vi "Reset.vi"(10 "Index":i32, 11 "Variables in":refnum<class "Variables.lvclass">) -> (3 "Variables out":refnum<class "Variables.lvclass">)   [LabVIEW 2020, in "VolatusSeq.lvlib" / "Variables.lvclass"]
uses:
  Variables.lvclass
  Variables.lvclass/Variables.ctl
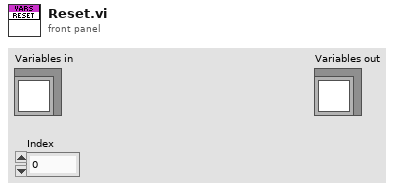
[diagram p1: front panel]
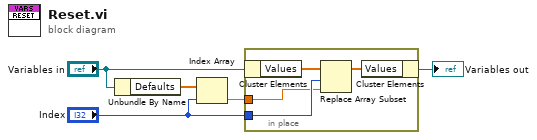
[diagram p0: block diagram]
diagram:
  n1 = Unbundle By Name("Variables in") -> ("Defaults"=w4:dbl[])
  n2 = Index Array(array=w4, index="Index") -> (element=w3:dbl)
  n3 = in-place {
    in-place-border: w3 -> [w7]
    in-place-border: "Index" -> [w8]
    n4 = in-place-cluster #1("Variables in") -> ("Values"=w9:dbl[])
    n5 = Replace Array Subset(array=w9, new element=w7, index=w8) -> (w6:dbl[])
    n6 = in-place-cluster #1("Values"=w6) -> (→"Variables out":refnum<class "Variables.lvclass">)
  }
